vi "Self-Test.vi"(8 "error in (no error)":errorcluster, 11 "VISA resource name":refnum<visa-resource-name>) -> (0 "error out":errorcluster, 1 "Self-Test Result Message":string, 2 "Self-Test Result Code":i32, 3 "VISA resource name out":refnum<visa-resource-name>)   [LabVIEW 2015, in "Template - DMM.lvlib"]
doc: "Runs the instrument's self-test routine and returns the test results."
uses:
  <instrlib>/_Template - DMM/Template - DMM.lvlib
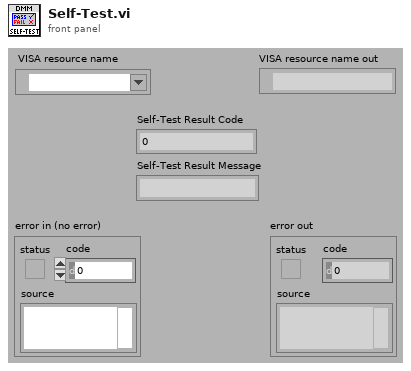
[diagram p1: front panel]
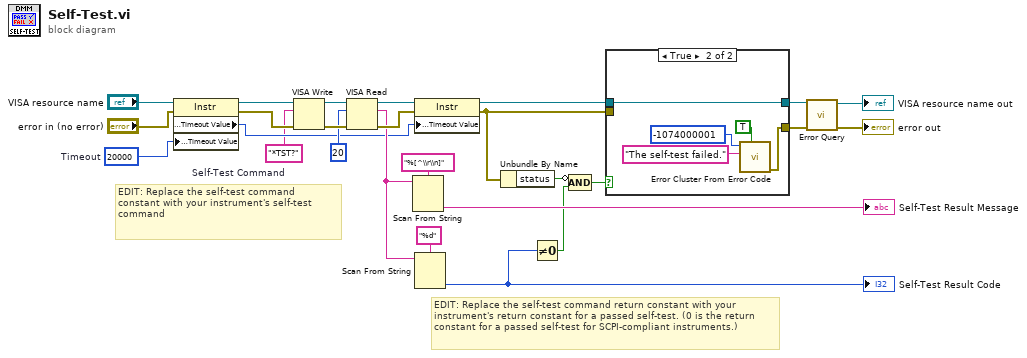
[diagram p0: block diagram]
diagram:
  w13 = u32 20000  # Timeout
  w9 = "*TST?"  # Self-Test Command
  # "EDIT: Replace the self-test command return constant with your instrument's return constant for a passed self-test. (0 is the return constant for a passed self-test for SCPI-compliant instruments.)"
  # "EDIT: Replace the self-test command constant with your instrument's self-test command"
  n1 = property class="Instr"(reference="VISA resource name", error in="error in (no error)", "General Settings:Timeout Value"=w13) -> (reference out=w11:refnum<visa-resource-name>, error out=w12:errorcluster, "General Settings:Timeout Value"=w10:u32)
  n2 = VISA Write(VISA resource name=w11, write buffer=w9, error in (no error)=w12) -> (VISA resource name out=w22:refnum<visa-resource-name>, error out=w21:errorcluster)  [unwired: 1 out]
  n3 = VISA Read(VISA resource name=w22, byte count=u32 20 ("byte count (20)"), error in (no error)=w21) -> (VISA resource name out=w24:refnum<visa-resource-name>, read buffer=w17:string, error out=w23:errorcluster)  [unwired: 1 out]
  n4 = Scan From String(format string="%[^\\r\\n]" ("Format String"), input string=w17) -> (output 1=→"Self-Test Result Message":string)  [unwired: 3 in, 3 out]
  n5 = property class="Instr"(reference=w24, error in=w23, "General Settings:Timeout Value"=w10) -> (reference out=w8:refnum<visa-resource-name>, error out=w7:errorcluster)
  n6 = Scan From String(format string="%d", input string=w17) -> (output 1=w1:i32)  [unwired: 3 in, 3 out]
  "Self-Test Result Code" <- w1
  n7 = Unbundle By Name(w7) -> ("status"=w3:bool)
  n8 = Not Equal To 0?(x=w1) -> (x != 0?=w4:bool)
  n9 = Compound Arithmetic op=AND(invert w3, w4) -> (w2:bool)
  n10 = case shown="True" w2 {
    tunnel: w8 -> [w28 w33]
    tunnel: w7 -> [w27 _]
    tunnel: [w27 w29] -> w6
    tunnel: [w28 w33] -> w5
    frame False {
    }
    frame True {
      n11 = call <vilib>:"Error Cluster From Error Code.vi"("show call chain? (False)"=TRUE, "error message (\"\")"="The self-test failed." ("Source (VI Name)"), "error code (0)"=-1074000001 ("Code")) -> ("error out"=w29:errorcluster)  [unwired: 6 in]
    }
  }
  n12 = call <instrlib>:"Error Query.vi"("error in (no error)"=w6, "VISA resource name"=w5) -> ("error out"=→"error out":errorcluster, "VISA resource name out"=→"VISA resource name out":refnum<visa-resource-name>)  [unwired: 6 in, 2 out]
